vi "字符串精度转换.vi"(9 "数组输入":string[](array[string]), 10 "数据精度":i32=6, 11 "输入字符串":string) -> (1 "数组输出":string[](array[string]), 3 "输出字符串":string)   [LabVIEW 2016, in "数据传输系统.lvlib"]
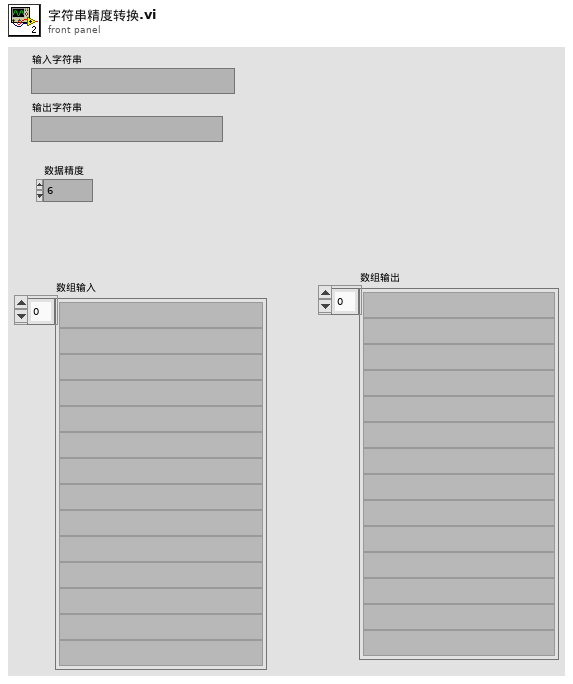
[diagram p1: front panel]
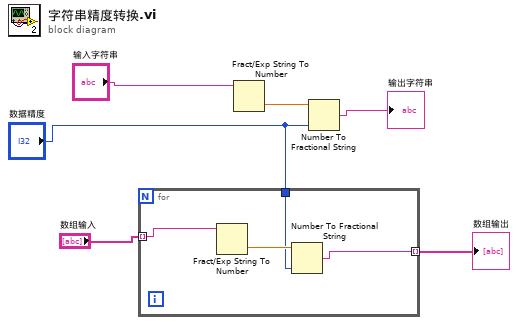
[diagram p0: block diagram]
diagram:
  n1 = for {
    tunnel: "数组输入" -> [w9] mode=indexing
    tunnel: [w8] -> w2 mode=indexing
    tunnel: "数据精度" -> [w7]
    n2 = Fract/Exp String To Number(string=w9) -> (number=w10:dbl)  [unwired: 3 in, 1 out]
    n3 = Number To Fractional String(number=w10, precision (6)=w7) -> (F-format string=w8:string)  [unwired: 2 in]
  }
  "数组输出" <- w2
  n4 = Fract/Exp String To Number(string="输入字符串") -> (number=w6:dbl)  [unwired: 3 in, 1 out]
  n5 = Number To Fractional String(number=w6, precision (6)="数据精度") -> (F-format string=→"输出字符串":string)  [unwired: 2 in]
